vi "BoundingBox.vi"(6 "Algorithm":enum16{"RRT", "A*"}(ring), 8 "k":i32=1, 9 "Depth":i32=1, 10 "Tree":dbl[][](array[numeric]), 11 "index":i32) -> (2 "Bounding Box":dbl[](array[numeric]))   [LabVIEW 2016]
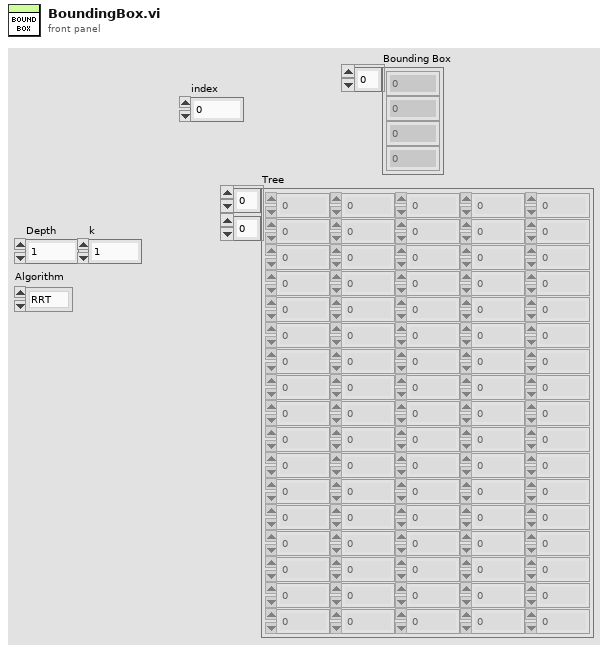
[diagram p1: front panel]
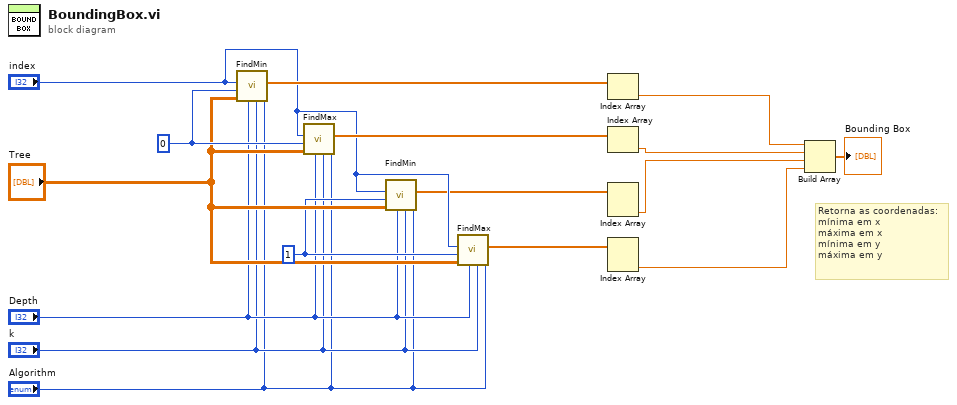
[diagram p0: block diagram]
diagram:
  w12 = 1 ("Dim")
  w16 = 0 ("Dim")
  # "Retorna as coordenadas:\nmínima em x\nmáxima em x\nmínima em y\nmáxima em y"
  n1 = call "FindMin.vi"("Algorithm"="Algorithm", "k"="k", "Depth"="Depth", "KD Tree"="Tree", "Dim"=w16, "index"="index") -> ("Min Node"=w14:dbl[])  [unwired: 5 in]
  n2 = call "FindMax.vi"("Algorithm"="Algorithm", "k"="k", "Depth"="Depth", "KD Tree"="Tree", "Dim"=w16, "index"="index") -> ("Max Node"=w15:dbl[])  [unwired: 5 in]
  n3 = call "FindMin.vi"("Algorithm"="Algorithm", "k"="k", "Depth"="Depth", "KD Tree"="Tree", "Dim"=w12, "index"="index") -> ("Min Node"=w7:dbl[])  [unwired: 5 in]
  n4 = call "FindMax.vi"("Algorithm"="Algorithm", "k"="k", "Depth"="Depth", "KD Tree"="Tree", "Dim"=w12, "index"="index") -> ("Max Node"=w6:dbl[])  [unwired: 5 in]
  n5 = Index Array(array=w14) -> (element=w5:dbl)  [unwired: 1 in]
  n6 = Index Array(array=w15) -> (element=w4:dbl)  [unwired: 1 in]
  n7 = Index Array(array=w7) -> (element #2=w3:dbl)  [unwired: 2 in, 1 out]
  n8 = Index Array(array=w6) -> (element #2=w2:dbl)  [unwired: 2 in, 1 out]
  n9 = Build Array(w5, w4, w3, w2) -> (→"Bounding Box":dbl[])
